vi "SetLabel.vi"(8 "Error In":errorcluster, 9 "Value":string, 10 "Label":string, 11 "reference in":refnum<class "UserManager.lvclass">) -> (0 "Error Out":errorcluster, 3 "reference in":refnum<class "UserManager.lvclass">)   [LabVIEW 2021]
uses:
  .Externals/Library_TAF_UserManager/UserManager/UserManager/UserManager.lvclass
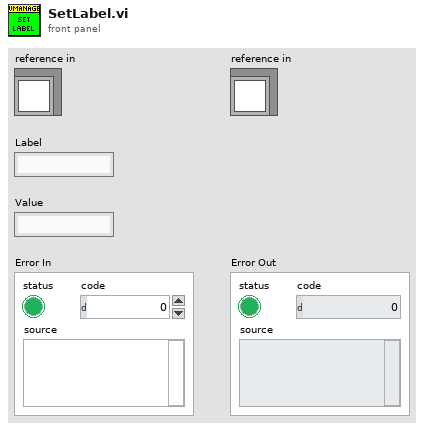
[diagram p1: front panel]
types:
  T1 = typedef "UserMananger.lvlib/UserManager.lvclass/ObjectAttributes.ctl" = cluster{"Interfaces":cluster{"ActivationUpdated":refnum<class "IAuthorizationUpdated.lvclass">}, "Locals":cluster{"MainGUIActive":refnum<queue>, "Evaluations":cluster{"Label":string, "Value":string}[]}, "Persistent":cluster{"Dummy":bool}}
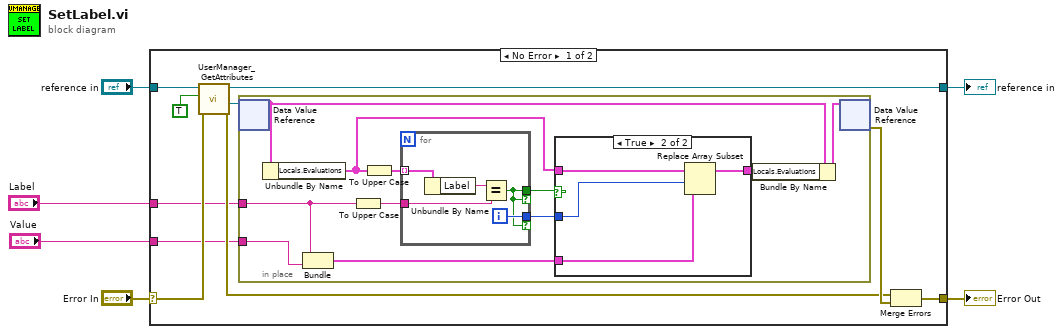
[diagram p0: block diagram]
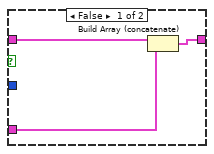
[diagram p2: hidden frame]
diagram:
  n1 = case shown="No Error" "Error In" {
    selector: "Error In" -> [w14 w41]
    tunnel: [w9 w41] -> w5
    tunnel: [w15 w40] -> w3
    tunnel: "reference in" -> [w16 w40]
    tunnel: "Label" -> [w8 _]
    tunnel: "Value" -> [w7 _]
    frame No Error {
      n2 = call "UserManager_GetAttributes.vi"("error in (no error)"=w14, "OnlyGetDvrReference(False)"=TRUE, "reference in"=w16) -> ("error out"=w10:errorcluster, "DataRef"=w11:refnum<data-value>, "reference out"=w15:refnum<class "UserManager.lvclass">)  [unwired: 5 in, 1 out]
      n3 = in-place {
        in-place-border: w8 -> [w21]
        in-place-border: w7 -> [w20]
        n4 = in-place-dvr #1(w11) -> (w26:T1)  [unwired: 1 out]
        n5 = Unbundle By Name(w26) -> ("Locals.Evaluations"=w17:cluster{"Label":string, "Value":string}[])
        n6 = Bundle("Label"=w21, "Value"=w20) -> (w19:cluster{"Label":string, "Value":string})  [unwired: 1 in]
        n7 = To Upper Case(1:w21) -> (0:w23:string)
        n8 = To Upper Case(1:w17) -> (0:w24:cluster{"Label":string, "Value":string}[])
        n9 = for {
          tunnel: w24 -> [w32] mode=indexing
          tunnel: w23 -> [w30]
          tunnel: [w28] -> w22 if=w28
          tunnel: [w29] -> w18 if=w28
          i -> [w29]
          n10 = Unbundle By Name(w32) -> ("Label"=w31:string)
          n11 = Equal?(x=w31, y=w30) -> (x = y?=w28:bool)
        }
        n12 = case shown="True" w22 {
          tunnel: w17 -> [w35 w39]
          tunnel: [w34 w38] -> w25
          tunnel: w19 -> [w33 w36]
          tunnel: w18 -> [_ w37]
          frame False {
            n13 = Build Array (concatenate)(w35, w33) -> (w34:cluster{"Label":string, "Value":string}[])
          }
          frame True {
            n14 = Replace Array Subset(array=w39, new element=w36, index=w37) -> (w38:cluster{"Label":string, "Value":string}[])
          }
        }
        n15 = Bundle By Name(cluster=w26, "Locals.Evaluations"=w25) -> (w27:T1)
        n16 = in-place-dvr #1(w27) -> (w12:errorcluster)  [unwired: 1 out]
      }
      n17 = Merge Errors(w10, w12) -> (w9:errorcluster)
    }
    frame Error {
    }
  }
  "Error Out" <- w5
  "reference in" <- w3
